vi "Configure Correction State.vi"(7 "Load Correction State (F:Disable)":bool, 8 "error in (no error)":errorcluster, 9 "Short Correction State (F:Disable)":bool, 10 "Open Correction State (F:Disable)":bool, 11 "VISA resource name":refnum<visa-resource-name>) -> (0 "error out":errorcluster, 3 "VISA resource name out":refnum<visa-resource-name>)   [LabVIEW 2016, in "Agilent E4980.lvlib"]
doc: "Configures the states for open, short and load corrections."
uses:
  <instrlib>/Agilent E4980/Agilent E4980.lvlib
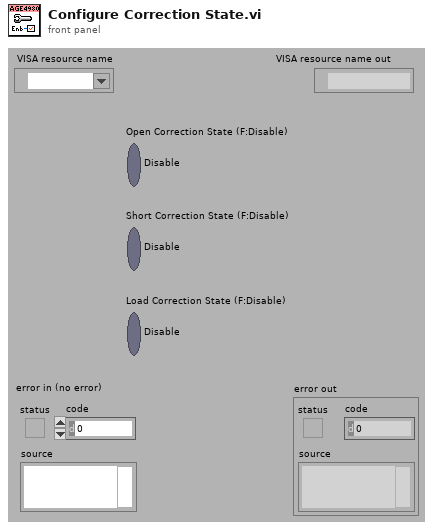
[diagram p1: front panel]
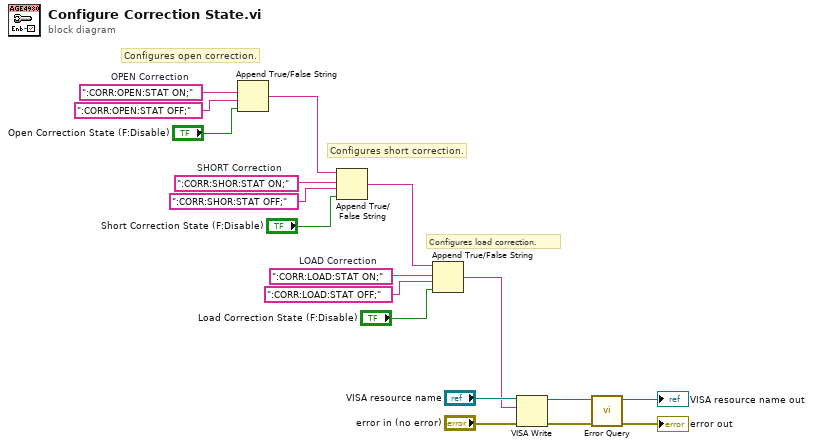
[diagram p0: block diagram]
diagram:
  w13 = ":CORR:LOAD:STAT ON;"  # LOAD Correction
  w16 = ":CORR:SHOR:STAT ON;"  # SHORT Correction
  w18 = ":CORR:OPEN:STAT ON;"  # OPEN Correction
  # "Configures load correction."
  # "Configures short correction."
  # "Configures open correction."
  n1 = Append True/False String(1:"Open Correction State (F:Disable)", 2:":CORR:OPEN:STAT OFF;" ("false string"), 3:w18) -> (0:w4:string)  [unwired: 1 in]
  n2 = Append True/False String(1:"Short Correction State (F:Disable)", 2:":CORR:SHOR:STAT OFF;" ("false string"), 3:w16, 4:w4) -> (0:w3:string)
  n3 = Append True/False String(1:"Load Correction State (F:Disable)", 2:":CORR:LOAD:STAT OFF;" ("false string"), 3:w13, 4:w3) -> (0:w2:string)
  n4 = VISA Write(VISA resource name="VISA resource name", write buffer=w2, error in (no error)="error in (no error)") -> (VISA resource name out=w8:refnum<visa-resource-name>, error out=w7:errorcluster)  [unwired: 1 out]
  n5 = call <instrlib>:"Error Query.vi"("error in (no error)"=w7, "VISA resource name"=w8) -> ("error out"=→"error out":errorcluster, "VISA resource name out"=→"VISA resource name out":refnum<visa-resource-name>)  [unwired: 6 in, 2 out]
